vi "Filter Clusters.vi"(8 "Error In":errorcluster, 11 "GObjects":refnum<vi>[](array[refnum])) -> (0 "Error Out":errorcluster, 3 "Clusters":refnum<vi>[](array[refnum]))   [LabVIEW 2017, in "Toolkit.lvlib"]
uses:
  Toolkit.lvlib
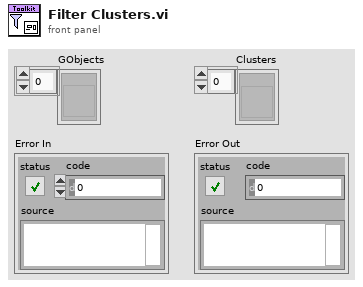
[diagram p1: front panel]
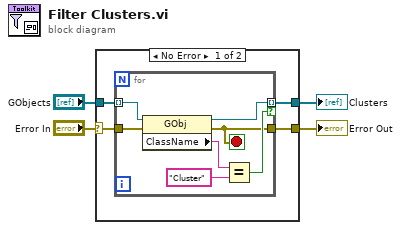
[diagram p0: block diagram]
diagram:
  n1 = case shown="No Error" "Error In" {
    selector: "Error In" -> [w7 w16]
    tunnel: "GObjects" -> [w8 _]
    tunnel: [w5 w16] -> w2
    tunnel: [w6 _] -> w1
    frame No Error {
      n2 = for {
        tunnel: w8 -> [w15] mode=indexing
        tunnel: w7 -> [w14]
        tunnel: [w11] -> w6 mode=indexing if=w10
        tunnel: [w9] -> w5
        stop <- w9 stop-if-true
        n3 = property class="GObj"(reference=w15, error in=w14) -> (reference out=w11:refnum<vi>, error out=w9:errorcluster, "ClassName"=w13:string)
        n4 = Equal?(x=w13, y="Cluster") -> (x = y?=w10:bool)
      }
    }
    frame Error {
    }
  }
  "Error Out" <- w2
  "Clusters" <- w1
